vi "stopTransport.vi"(8 "error in (no error)":errorcluster, 11 "Inst.Transport in":refnum<class "Inst.Transport.lvclass">) -> (0 "error out":errorcluster, 3 "Inst.Transport out":refnum<class "Inst.Transport.lvclass">)   [LabVIEW 2019, in "Inst.Transport.lvclass"]
uses:
  Inst.Transport.lvclass
  Typedefs/Inst.Transport.PublicCommands--Enum.ctl
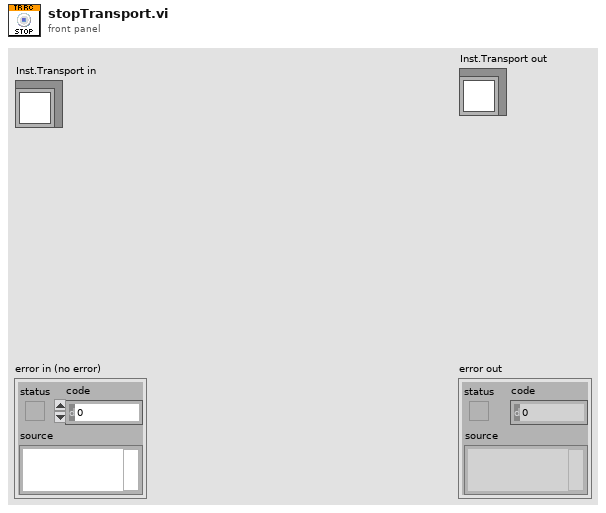
[diagram p1: front panel]
types:
  T1 = typedef "Inst.Transport.lvclass/Inst.Transport.PublicCommands--Enum.ctl" = enum16{"startTransport", "stopTransport", "getStatus", "setExptFolder", "getExptFolder", "setExptComments", "getExptComments", "setExptParam", "appendExptParam", "clearExptParam", "setSweepConfig", "getSweepConfig", "setRefreshTime"}
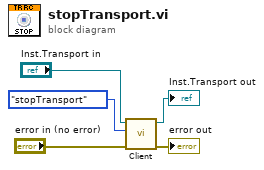
[diagram p0: block diagram]
diagram:
  n1 = call-dynamic "Client.vi"("error in (no error)"="error in (no error)", "Command in"=Inst.Transport.PublicCommands--Enum."stopTransport" ("Commands"), "Instrument in"="Inst.Transport in") -> ("error out"=→"error out":errorcluster, "Instrument out"=→"Inst.Transport out":refnum<class "Inst.Transport.lvclass">)  [unwired: 5 in, 2 out]
